vi "Find Firmware Path.vi"(8 "error in":errorcluster, 11 "Product Name":string) -> (0 "error out":errorcluster, 2 "Path Found?":bool, 3 "Firmware Path":path)   [LabVIEW 2020]
doc: "Retrieves the firmware path according to the cRIO model."
uses:
  <vilib>/Utility/sysdir.llb/System Directory Type.ctl
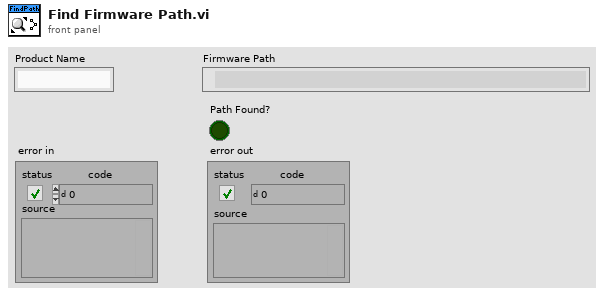
[diagram p1: front panel]
types:
  T1 = typedef "System Directory Type.ctl" = i32
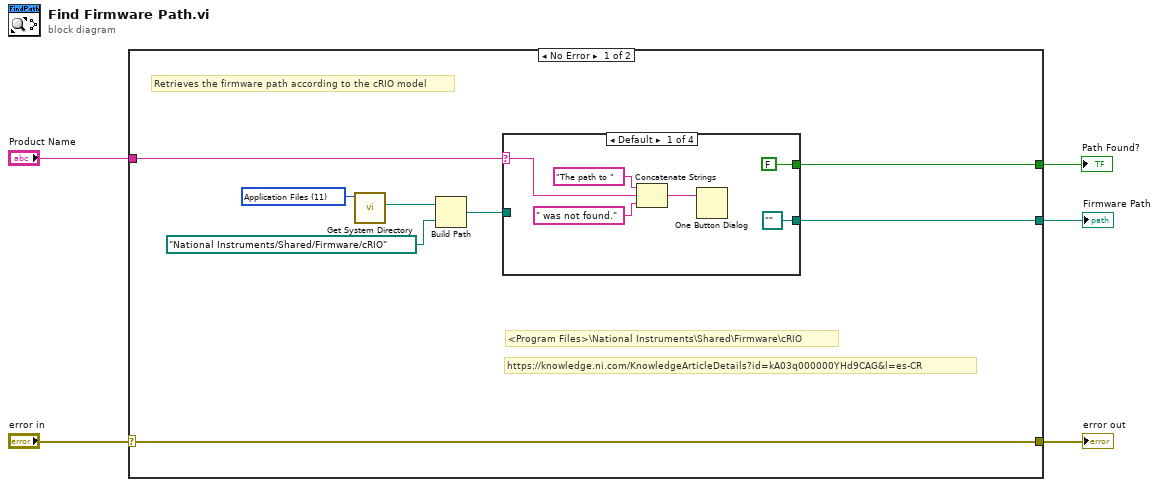
[diagram p0: block diagram]
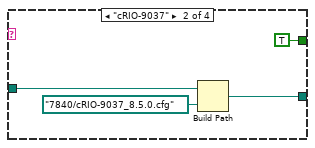
[diagram p2: hidden frame]
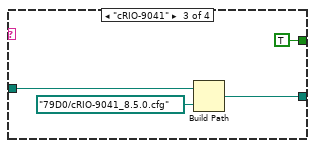
[diagram p3: hidden frame]
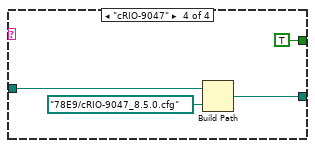
[diagram p4: hidden frame]
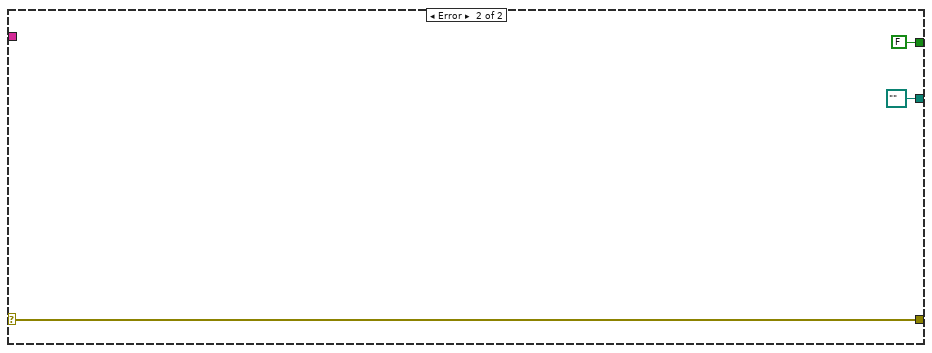
[diagram p5: hidden frame]
diagram:
  n1 = case shown="No Error" "error in" {
    selector: "error in" -> [w7 w34]
    tunnel: [w13 path "" ("appended path")] -> w5
    tunnel: "Product Name" -> [w8 _]
    tunnel: [w7 w34] -> w2
    tunnel: [w6 FALSE] -> w1
    frame No Error {
      w9 = T1 11 items=["User Home"=0, "User Desktop"=1, "User Documents"=2, "User Application Data"=3, "User Preferences"=4, "User Temporary"=5, "Public Documents"=6, "Public Application Data"=7, "Public Preferences"=8, "Public Cache"=13, "System Core Libraries"=9, "System Installed Libraries"=10, "Application Files"=11, "Boot Volume Root"=12] ("system directory type")
      # "Retrieves the firmware path according to the cRIO model"
      # "https://knowledge.ni.com/KnowledgeArticleDetails?id=kA03q000000YHd9CAG&l=es-CR"
      # "<Program Files>\\National Instruments\\Shared\\Firmware\\cRIO"
      n2 = call <vilib>:"Get System Directory.vi"("system directory type"=w9) -> ("system directory"=w10:path)  [unwired: 10 in]
      n3 = Build Path(base path=w10, name or relative path=path "National Instruments/Shared/Firmware/cRIO") -> (appended path=w12:path)
      n4 = case shown="Default" w8 {
        selector: w8 -> [w17 _ _ _]
        tunnel: w12 -> [_ w23 w26 w30]
        tunnel: [path "" ("appended path") w21 w25 w29] -> w13
        tunnel: [FALSE TRUE TRUE TRUE] -> w6
        frame Default {
          n5 = Concatenate Strings("The path to ", w17, " was not found.") -> (w15:string)
          n6 = One Button Dialog(message=w15) -> ()  [unwired: 1 in, 1 out]
        }
        frame "cRIO-9037" {
          n7 = Build Path(base path=w23, name or relative path=path "7840/cRIO-9037_8.5.0.cfg") -> (appended path=w21:path)
        }
        frame "cRIO-9041" {
          n8 = Build Path(base path=w26, name or relative path=path "79D0/cRIO-9041_8.5.0.cfg") -> (appended path=w25:path)
        }
        frame "cRIO-9047" {
          n9 = Build Path(base path=w30, name or relative path=path "78E9/cRIO-9047_8.5.0.cfg") -> (appended path=w29:path)
        }
      }
    }
    frame Error {
    }
  }
  "Firmware Path" <- w5
  "error out" <- w2
  "Path Found?" <- w1
